vi "readcoefficientsettings.vi"(2 "Path":path, 3 "error in (no error)":errorcluster) -> (5 "Path 2":path, 6 "?":T1, 7 "error out":errorcluster)   [LabVIEW 2012]
uses:
  <vilib>/Utility/config.llb/Read Key (Double).vi
  <vilib>/Utility/config.llb/NI_LVConfig.lvlib
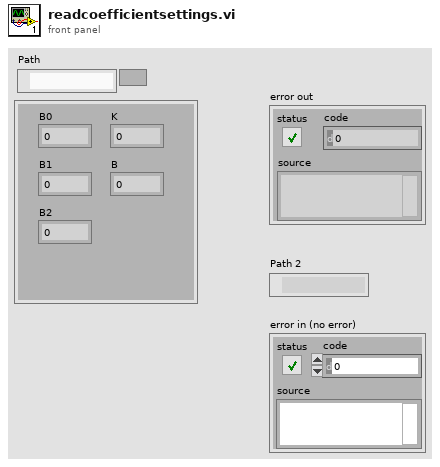
[diagram p1: front panel]
types:
  T1 = cluster{"B0":dbl, "B1":dbl, "B2":dbl, "K":dbl, "B":dbl}
  T2 = typedef "NI_LVConfig.lvlib/Config Data RefNum.ctl" = refnum<k1>
  T3 = cluster{"value":dbl, "value":dbl, "value":dbl, "value":dbl, "value":dbl}
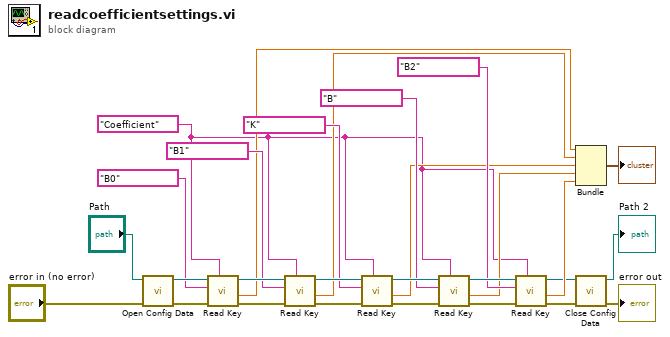
[diagram p0: block diagram]
diagram:
  w2 = "Coefficient"
  n1 = call <vilib>:"Open Config Data.vi"("error in (no error)"="error in (no error)", "configuration file path"="Path") -> ("error out"=w22:errorcluster, "refnum"=w27:T2)  [unwired: 7 in, 1 out]
  n2 = call-poly <vilib>:"Read Key.vi"("section"=w2, "error in (no error)"=w22, "key"="B0", "refnum"=w27) -> ("error out"=w21:errorcluster, "value"=w7:dbl, "refnum out"=w26:T2)  [unwired: 4 in, 1 out]
  n3 = call-poly <vilib>:"Read Key.vi"("section"=w2, "error in (no error)"=w21, "key"="B1", "refnum"=w26) -> ("error out"=w20:errorcluster, "value"=w8:dbl, "refnum out"=w25:T2)  [unwired: 4 in, 1 out]
  n4 = call-poly <vilib>:"Read Key.vi"("section"=w2, "error in (no error)"=w20, "key"="K", "refnum"=w25) -> ("error out"=w19:errorcluster, "value"=w9:dbl, "refnum out"=w24:T2)  [unwired: 4 in, 1 out]
  n5 = call-poly <vilib>:"Read Key.vi"("section"=w2, "error in (no error)"=w19, "key"="B", "refnum"=w24) -> ("error out"=w18:errorcluster, "value"=w10:dbl, "refnum out"=w23:T2)  [unwired: 4 in, 1 out]
  n6 = call-poly <vilib>:"Read Key.vi"("section"=w2, "error in (no error)"=w18, "key"="B2", "refnum"=w23) -> ("error out"=w3:errorcluster, "value"=w11:dbl, "refnum out"=w4:T2)  [unwired: 4 in, 1 out]
  n7 = Bundle("value"=w7, "value"=w8, "value"=w9, "value"=w10, "value"=w11) -> (→"?":T3)  [unwired: 1 in]
  n8 = call <vilib>:"Close Config Data.vi"("error in (no error)"=w3, "refnum"=w4) -> ("error out"=→"error out":errorcluster, "file path"=→"Path 2":path)  [unwired: 8 in]
